vi "Offset Calculation.vi"(8 "error in (no error)":errorcluster, 9 "Voltage@20A":dbl, 10 "Voltage@10A":dbl, 11 "Voltage@0.1A":dbl) -> (0 "error out":errorcluster, 3 "Voltage Offset":dbl)   [LabVIEW 2025]
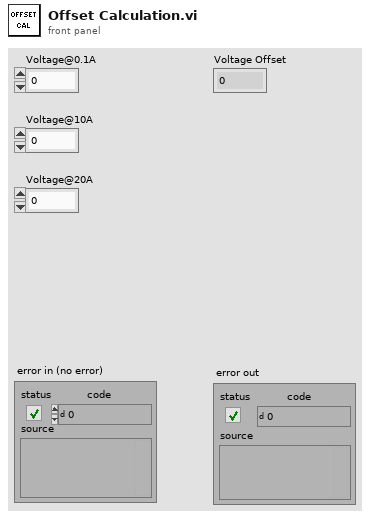
[diagram p1: front panel]
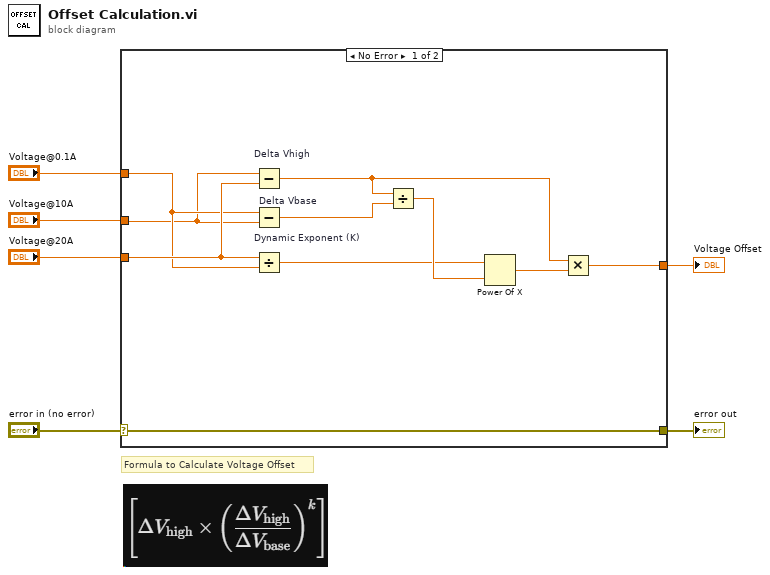
[diagram p0: block diagram]
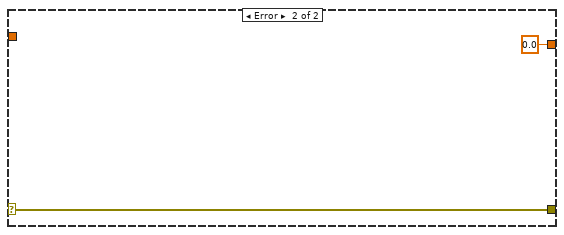
[diagram p2: hidden frame]
diagram:
  # "Formula to Calculate Voltage Offset"
  n1 = case shown="No Error" "error in (no error)" {
    selector: "error in (no error)" -> [w10 w18]
    tunnel: "Voltage@20A" -> [w9 _]
    tunnel: "Voltage@10A" -> [w7 _]
    tunnel: "Voltage@0.1A" -> [w8 _]
    tunnel: [w11 0.0] -> w2
    tunnel: [w10 w18] -> w1
    frame No Error {
      n2 = Subtract "Delta Vhigh"(x=w7, y=w9) -> (x-y=w12:dbl)
      n3 = Subtract "Delta Vbase"(x=w8, y=w7) -> (x-y=w16:dbl)
      n4 = Divide "Dynamic Exponent (K)"(x=w9, y=w8) -> (x/y=w14:dbl)
      n5 = Divide(x=w12, y=w16) -> (x/y=w15:dbl)
      n6 = Power Of X(1:w15, 2:w14) -> (0:w13:dbl)
      n7 = Multiply(x=w12, y=w13) -> (x*y=w11:dbl)
    }
    frame Error {
    }
  }
  "error out" <- w1
  "Voltage Offset" <- w2
